vi "zad3Cieslikiewicz.vi"() -> ()   [LabVIEW 2020]
panel:
  in  "Numeric":dbl=1.0 min=1.0 max=4.0 step=1.0
  in  "stop":bool
  out "Boolean 4":bool
  out "Boolean 3":bool
  out "Boolean 2":bool
  out "Boolean":bool
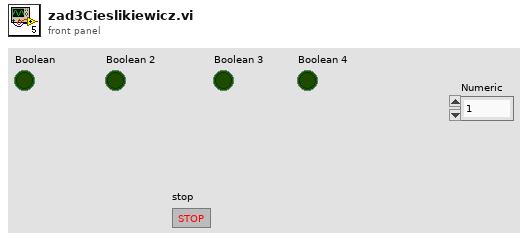
[diagram p1: front panel]
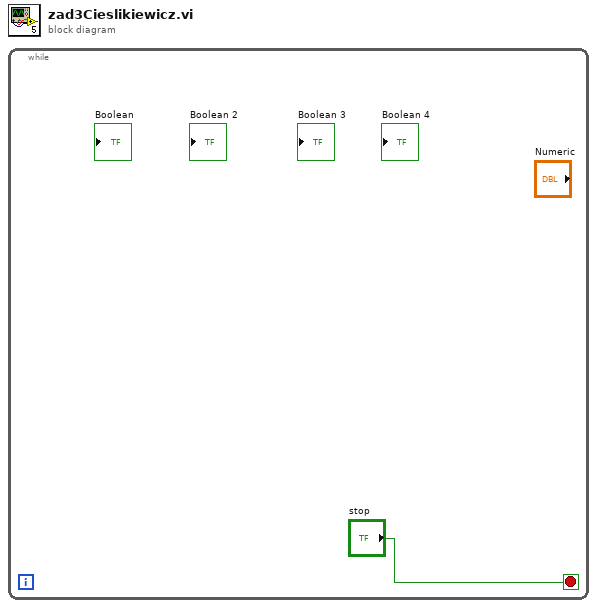
[diagram p0: block diagram]
diagram:
  n1 = while {
    stop <- "stop" stop-if-true
  }
